vi "SVT UFF58 Write Generic.vi"(0 "file refnum":refnum<k20>, 1 "ID lines (1-3)":T3, 2 "data precision (double-precision:1)":T1=1 items=["single-precision", "double-precision"], 3 "function type":T2, 7 "ordinate values (Y Real)":dbl[](array[numeric]), 9 "ordinate values (Y Im)":dbl[](array[numeric]), 11 "error in (no error)":errorcluster, 12 "abscissa minimum (x0)":dbl, 13 "abscissa increment (dx)":dbl) -> (4 "dup file refnum":refnum<k20>, 6 "function refnum":refnum<k20>, 15 "error out":errorcluster)   [LabVIEW 2017, in "SoundVib_UFF58.lvlib"]
doc: "Writes data to the UFF58 (universal file format) file specified by the <B>file refnum</B> input. This VI also writes the fields in records 1, 2, and 3, <B>ID lines (1-3)</B>. You can write a single time domain waveform, multiple time domain waveforms, a single real frequency spectrum, multiple real frequency spectra, a single complex frequency spectrum, multiple complex frequency spectra, or generic data to a UFF file. If a frequency spectrum is in decibels, this VI converts the spectrum to linear before writing to the UFF58 file. The default instance, SVT UFF58 Write Time Waveform (1 Ch), writes a single time domain waveform to the file specified by the <B>file refnum</B> input. Wire data to the <B>file refnum</B> input to determine the polymorphic instance to use or manually select the instance."
uses:
  <vilib>/addons/Sound and Vibration/svt_UFF58/SoundVib_UFF58.lvlib
  <vilib>/addons/Sound and Vibration/svt_UFF58/subVIs/sv_IDLines123.ctl
  <vilib>/addons/Sound and Vibration/svt_UFF58/subVIs/sv_FunctionType.ctl
  <vilib>/addons/Sound and Vibration/svt_UFF58/subVIs/sv_UFF58 Data Precision.ctl
  <vilib>/addons/Sound and Vibration/svt_UFF58/subVIs/sv_UFF58 Check Data Valid (Generic).vi
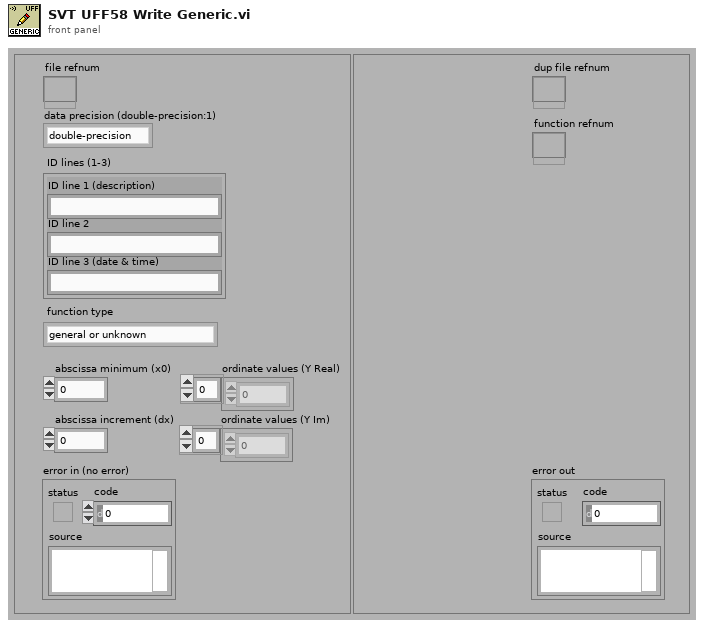
[diagram p1: front panel]
types:
  T1 = typedef "SoundVib_UFF58.lvlib/sv_UFF58 Data Precision.ctl" = u32
  T2 = typedef "SoundVib_UFF58.lvlib/sv_FunctionType.ctl" = enum16{"general or unknown", "time response", "auto spectrum", "cross spectrum", "frequency response function", "transmissibility", "coherence", "auto correlation", "cross correlation", "power spectral density (PSD)", "energy spectral density (ESD)", "probability density function", "spectrum", "cumulative frequency distribution", "peaks valley", "stress/cycles", "strain/cycles", "orbit", "mode indicator function", "force pattern", "partial power", "partial coherence", "eigenvalue", "eigenvector", "shock response spectrum", "finite impulse response filter", "multiple coherence", "order function", "phase compensation"}
  T3 = typedef "SoundVib_UFF58.lvlib/sv_IDLines123.ctl" = cluster{"ID line 1 (description)":string, "ID line 2":string, "ID line 3 (date & time)":string}
  T4 = typedef "SoundVib_UFF58.lvlib/sv_UFF58 DOF.ctl" = cluster{"function type":T2, "function ID number":i32, "version number":i32, "load case ID number":i32, "response entity name":string, "response node":i32, "response direction":T5, "reference entity name":string, "reference node":i32, "reference direction":T5}
  T5 = typedef "SoundVib_UFF58.lvlib/sv_UFF58 Response Direction.ctl" = i32
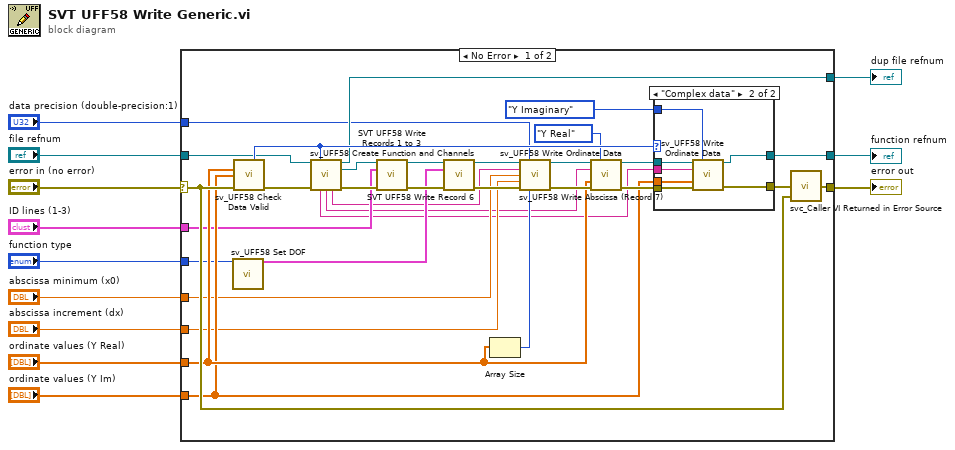
[diagram p0: block diagram]
diagram:
  n1 = case shown="No Error" "error in (no error)" {
    selector: "error in (no error)" -> [w23 w55]
    tunnel: [w24 w55] -> w12
    tunnel: "ID lines (1-3)" -> [w17 _]
    tunnel: [w33 w54] -> w10
    tunnel: "file refnum" -> [w41 w54]
    tunnel: "function type" -> [w18 _]
    tunnel: [w30 _] -> w2
    tunnel: "ordinate values (Y Real)" -> [w22 _]
    tunnel: "abscissa increment (dx)" -> [w20 _]
    tunnel: "abscissa minimum (x0)" -> [w19 _]
    tunnel: "ordinate values (Y Im)" -> [w21 _]
    tunnel: "data precision (double-precision:1)" -> [w13 _]
    frame No Error {
      n2 = call <vilib>:"sv_UFF58 Set DOF.vi"("function type"=w18) -> ("DOF identification (record 6)"=w34:T4)  [unwired: 14 in]
      n3 = call-poly <vilib>:"sv_UFF58 Check Data Valid.vi"("ordinate values (Y Real)"=w22, "ordinate values (Y Im)"=w21, "error in (no error)"=w23) -> ("real or complex data?"=w44:enum16{"Real data", "Complex data"}, "error out"=w29:errorcluster)  [unwired: 9 in, 2 out]
      n4 = call <vilib>:"sv_UFF58 Create Function and Channels.vi"("file refnum"=w41, "real or complex data?"=w44, "error in (no error)"=w29) -> ("dup file refnum"=w33:refnum<k20>, "function refnum"=w40:refnum<k20>, "ordinate denominator channel name"=w14:string, "ordinate numerator channel name"=w15:string, "abscissa channel name"=w16:string, "error out"=w39:errorcluster)  [unwired: 6 in, 1 out]
      n5 = call <vilib>:"SVT UFF58 Write Records 1 to 3.vi"("function refnum"=w40, "ID lines (1-3)"=w17, "error in (no error)"=w39) -> ("dup function refnum"=w43:refnum<k20>, "error out"=w42:errorcluster)  [unwired: 11 in]
      n6 = call <vilib>:"SVT UFF58 Write Record 6.vi"("function refnum"=w43, "DOF identification"=w34, "error in (no error)"=w42) -> ("dup function refnum"=w37:refnum<k20>, "error out"=w38:errorcluster)  [unwired: 11 in]
      n7 = Array Size(array=w22) -> (size(s)=w28:i32)
      n8 = call <vilib>:"sv_UFF58 Write Abscissa (Record 7).vi"("function refnum"=w37, "data precision (double-precision:1)"=w13, "Name"=w16, "x0"=w19, "dx"=w20, "error in (no error)"=w38, "channel length"=w28) -> ("dup function refnum"=w35:refnum<k20>, "error out"=w36:errorcluster)  [unwired: 7 in]
      n9 = call <vilib>:"sv_UFF58 Write Ordinate Data.vi"("function refnum"=w35, "channel to write"=enum16{"X", "Y Real", "Y Imaginary"}."Y Real", "ordinate channel name"=w15, "ordinate data"=w22, "error in (no error)"=w36) -> ("dup function refnum"=w31:refnum<k20>, "error out"=w32:errorcluster)  [unwired: 9 in]
      n10 = case shown="\"Complex data\"" w44 {
        tunnel: w32 -> [w46 w53]
        tunnel: w31 -> [w45 w52]
        tunnel: [w45 w51] -> w30
        tunnel: enum16{"X", "Y Real", "Y Imaginary"}."Y Imaginary" ("channel to write") -> [_ w50]
        tunnel: [w46 w49] -> w25
        tunnel: w21 -> [_ w48]
        tunnel: w14 -> [_ w47]
        frame "Real data", Default {
        }
        frame "Complex data" {
          n11 = call <vilib>:"sv_UFF58 Write Ordinate Data.vi"("function refnum"=w52, "channel to write"=w50, "ordinate channel name"=w47, "ordinate data"=w48, "error in (no error)"=w53) -> ("dup function refnum"=w51:refnum<k20>, "error out"=w49:errorcluster)  [unwired: 9 in]
        }
      }
      n12 = call <vilib>:"svc_Caller VI Returned in Error Source.vi"("warning input to caller"=w23, "error in (no error)"=w25) -> ("error out"=w24:errorcluster)  [unwired: 3 in]
    }
    frame Error {
    }
  }
  "dup file refnum" <- w10
  "error out" <- w12
  "function refnum" <- w2
